vi "RT Driver VI.vi"(7 "Operation":T1, 11 "Device Reference in":T2 format="%.0x") -> (0 "Error Code":i32)   [LabVIEW 2017, in "Data Sharing Framework Engine.lvlib"]
uses:
  Data Sharing Framework Engine.lvlib
  <vilib>/NI Veristand/Custom Device API/Custom Device Item Ref.ctl
  <vilib>/NI Veristand/Custom Device API/Hardware Interface Driver VI Operation.ctl
  VeriStand Framework/VeriStand Framework.lvclass
  <vilib>/NI Veristand/Custom Device API/Custom Device API.lvlib
  <vilib>/NI Veristand/Custom Device API/Custom Device Channel Type.ctl
  <vilib>/NI Veristand/Custom Device API/Data Access Type.ctl
  dsf core/Built/DSF.Engine.lvlibp/Engine/Classes/Framework/DSF.Engine.Framework.lvclass
  C:/Git/DSF/dsf core/Built/DSF.Engine.lvlibp/Engine/Classes/Framework/DSF.Engine.Framework.lvclass
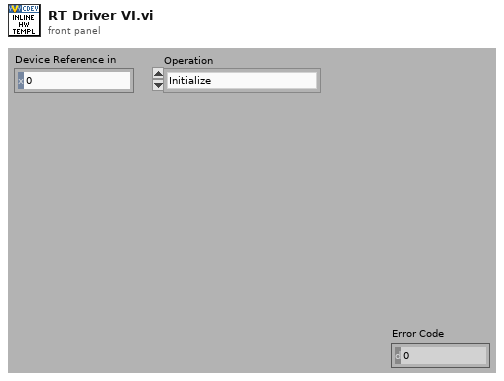
[diagram p1: front panel]
types:
  T1 = typedef "Custom Device API.lvlib/Hardware Interface Driver VI Operation.ctl" = enum16{"Initialize", "Start", "Read Data from HW", "Write Data to HW", "Close"}
  T2 = typedef "Custom Device API.lvlib/Custom Device Item Ref.ctl" = u64
  T3 = typedef "Custom Device API.lvlib/Custom Device Channel Type.ctl" = enum16{"Input", "Output"}
  T4 = typedef "Custom Device API.lvlib/Data Access Type.ctl" = enum16{"Read", "Write"}
  T5 = typedef "Custom Device API.lvlib/Data Reference.ctl" = i32
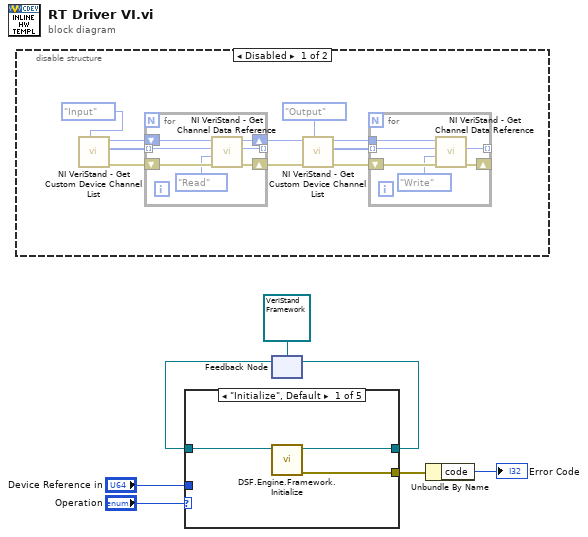
[diagram p0: block diagram]
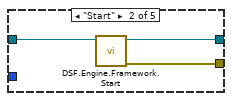
[diagram p2: hidden frame]
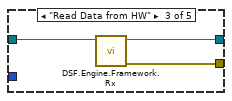
[diagram p3: hidden frame]
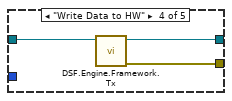
[diagram p4: hidden frame]
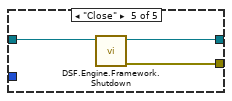
[diagram p5: hidden frame]
diagram:
  n1 = disable-structure shown="Disabled" {
    frame Disabled {
      n2 = call <vilib>:"NI VeriStand - Get Custom Device Channel List.vi"("Channel Type"=Custom_Device_Channel_Type."Input") -> ("error out"=w11:errorcluster, "Specified Channel Ref List"=w12:T2[], "Device Ref out"=w10:T2)  [unwired: 2 in, 6 out]
      n3 = for {
        shift-right: [w25] -> w15
        shift-left: w10 -> [w29]
        tunnel: w12 -> [w28] mode=indexing
        shift-right: [w26] -> w16
        shift-left: w11 -> [w30]
        tunnel: [w24] -> _ mode=indexing
        n4 = call <vilib>:"NI VeriStand - Get Channel Data Reference.vi"("error in (no error)"=w30, "Access"=Data_Access_Type."Read", "Channel Ref in"=w28, "Device Ref in"=w29) -> ("error out"=w26:errorcluster, "Channel Data Reference"=w24:T5, "Device Ref out"=w25:T2)  [unwired: 5 out]
      }
      n5 = call <vilib>:"NI VeriStand - Get Custom Device Channel List.vi"("Channel Type"=Custom_Device_Channel_Type."Output", "error in (no error)"=w16, "Device Ref in"=w15) -> ("error out"=w13:errorcluster, "Specified Channel Ref List"=w17:T2[], "Device Ref out"=w14:T2)  [unwired: 6 out]
      n6 = for {
        tunnel: w17 -> [w21] mode=indexing
        shift-right: [w19] -> _
        shift-left: w13 -> [w23]
        tunnel: [w18] -> _ mode=indexing
        tunnel: w14 -> [w22]
        n7 = call <vilib>:"NI VeriStand - Get Channel Data Reference.vi"("error in (no error)"=w23, "Access"=Data_Access_Type."Write", "Channel Ref in"=w21, "Device Ref in"=w22) -> ("error out"=w19:errorcluster, "Channel Data Reference"=w18:T5)  [unwired: 6 out]
      }
    }
    frame Enabled {
    }
  }
  n8 = feedback #1(refnum<class "VeriStand Framework.lvclass"> refnum ("Data Sharing Framework Engine.lvlib:VeriStand Framework.lvclass")) -> (w5:refnum<class "VeriStand Framework.lvclass">)
  n9 = case shown="\"Initialize\", Default" "Operation" {
    tunnel: [w33 w35 w38 w41 w44] -> w6
    tunnel: w5 -> [w31 w36 w39 w42 w45]
    tunnel: "Device Reference in" -> [_ _ _ _ _]
    tunnel: [w32 w34 w37 w40 w43] -> w3
    frame "Initialize", Default {
      n10 = call "DSF.Engine.Framework.Initialize.vi"("Framework type"=w31) -> ("error out"=w32:errorcluster, "Framework out"=w33:refnum<class "VeriStand Framework.lvclass">)  [unwired: 9 in]
    }
    frame "Start" {
      n11 = call "DSF.Engine.Framework.Start.vi"("Framework in"=w36) -> ("error out"=w34:errorcluster, "Framework out"=w35:refnum<class "VeriStand Framework.lvclass">)  [unwired: 9 in]
    }
    frame "Read Data from HW" {
      n12 = call "DSF.Engine.Framework.Rx.vi"("Framework in"=w39) -> ("error out"=w37:errorcluster, "Framework out"=w38:refnum<class "VeriStand Framework.lvclass">)  [unwired: 9 in]
    }
    frame "Write Data to HW" {
      n13 = call "DSF.Engine.Framework.Tx.vi"("Framework in"=w42) -> ("error out"=w40:errorcluster, "Framework out"=w41:refnum<class "VeriStand Framework.lvclass">)  [unwired: 9 in]
    }
    frame "Close" {
      n14 = call "DSF.Engine.Framework.Shutdown.vi"("Framework in"=w45) -> ("error out"=w43:errorcluster, "Framework out"=w44:refnum<class "VeriStand Framework.lvclass">)  [unwired: 9 in]
    }
  }
  n15 = feedback-in #1(w6) -> ()
  n16 = Unbundle By Name(w3) -> ("code"=→"Error Code":i32)
